vi "Initialize Front Panel.vi"(8 "error in (no error)":errorcluster, 11 "LeakyViewable in":refnum<class "LeakyViewable.lvclass">) -> (0 "error out":errorcluster, 3 "LeakyViewable out":refnum<class "LeakyViewable.lvclass">)   [LabVIEW 2015, in "ViewableDoubles.lvlib" / "LeakyViewable.lvclass"]
doc: "<License>\nCopyright © 2017 Composed Systems, LLC | All rights reserved\nwww.composed.io\n\nAuthor: Ethan Stern <ethan.stern@composed.io>\n\nThis software is provided \"AS IS\" WITHOUT WARRANTIES, either express or implied, AND IS FOR EDUCATIONAL PURPOSES ONLY.\n</License>"
uses:
  LeakyViewable.lvclass
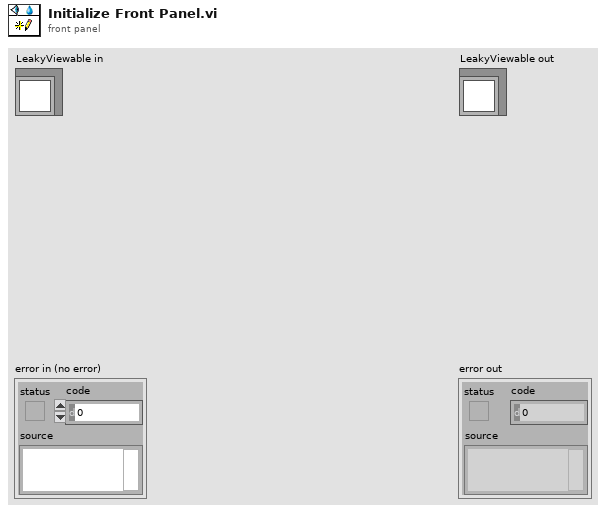
[diagram p1: front panel]
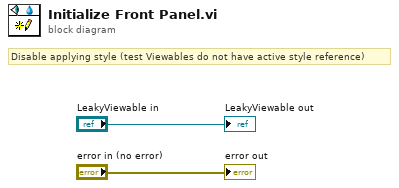
[diagram p0: block diagram]
diagram:
  # "Disable applying style (test Viewables do not have active style reference)"
  "error out" <- "error in (no error)"
  "LeakyViewable out" <- "LeakyViewable in"
